vi "VariantFacade.vi"(0 "Data In":T6, 2 "Display State In":T2, 3 "Container State":T5) -> (6 "Data Out":T6, 7 "Display State Out":T2, 8 "Action":T1)   [LabVIEW 2011, in "VariantXControl__VP.xctl"]
uses:
  VariantXControl__VP.xctl
  VariantData.ctl
  <vilib>/_xctls/Container State.ctl
  VariantState.ctl
  Permissions.ctl
  TreeSettings.ctl
  <vilib>/_xctls/Action.ctl
  <userlib>/_OpenG.lib/comparison/comparison.llb/Variant Changed__ogtk.vi
  <vilib>/_xctls/XControlSupport.lvlib
panel:
  in  "VariantTree":string(tree)
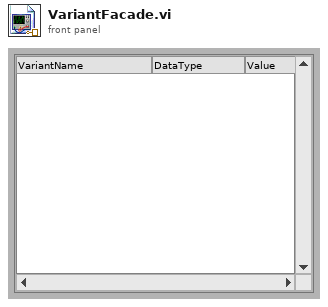
[diagram p1: front panel]
types:
  T1 = typedef "XControlSupport.lvlib/Action.ctl" = cluster{"Data Changed?":bool, "State Changed?":bool, "Action Name":string}
  T2 = typedef "VariantXControl__VP.xctl/VariantState.ctl" = cluster{"State":string, "Messages":cluster{"Message":string, "Parameter":variant}[], "Current run":i32, "Start run":i32, "LastTag":string, "Tags":string[], "Length":i32, "Permissions":T3, "IsProbe?":bool, "Changed":bool, "TreeSettings":T4, "Tree Ref":refnum<vi>}
  T3 = typedef "VariantXControl__VP.xctl/Permissions.ctl" = cluster{"Reset":bool, "TraverseAttributes":bool, "Colorize":bool}
  T4 = typedef "VariantXControl__VP.xctl/TreeSettings.ctl" = cluster{"Traverse":bool, "Colorize":bool}
  T5 = typedef "XControlSupport.lvlib/Container State.ctl" = cluster{"Indicator?":bool, "Run Mode?":bool, " Refnum":refnum<vi>}
  T6 = typedef "VariantXControl__VP.xctl/VariantData.ctl" = variant
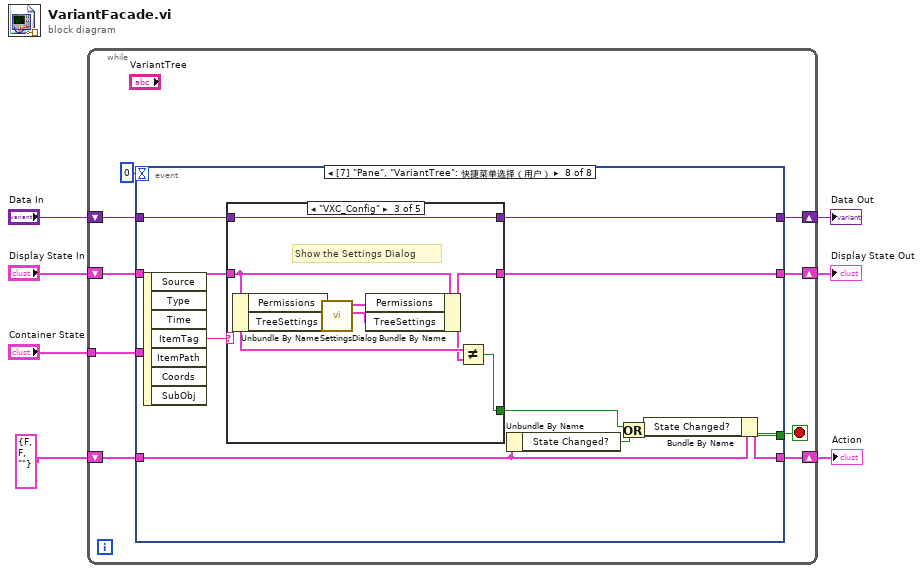
[diagram p0: block diagram]
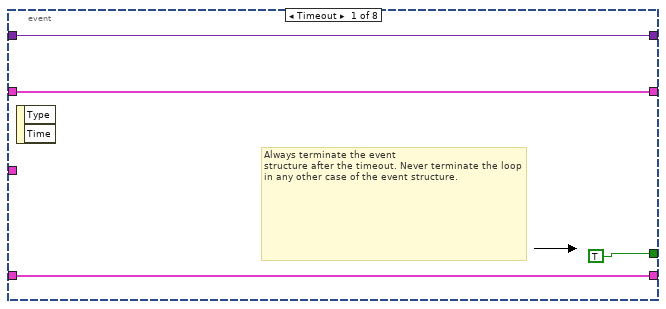
[diagram p2: hidden frame]
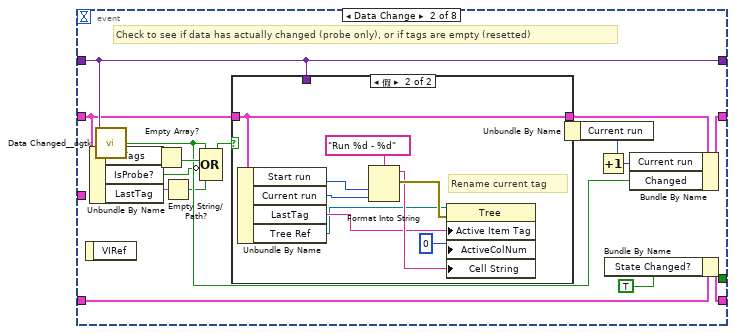
[diagram p3: hidden frame]
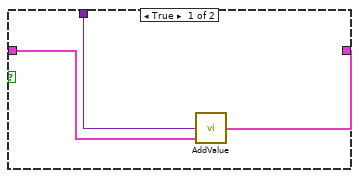
[diagram p4: hidden frame]
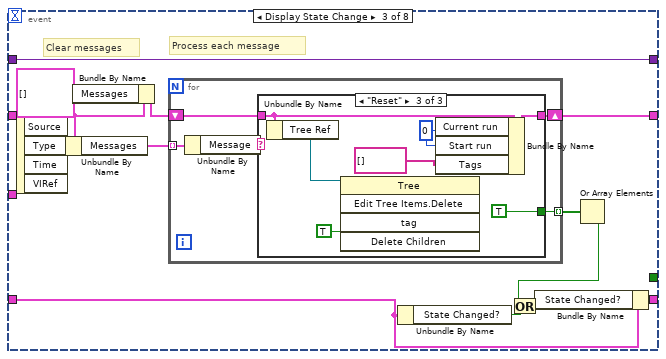
[diagram p5: hidden frame]
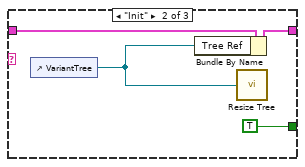
[diagram p7: hidden frame]
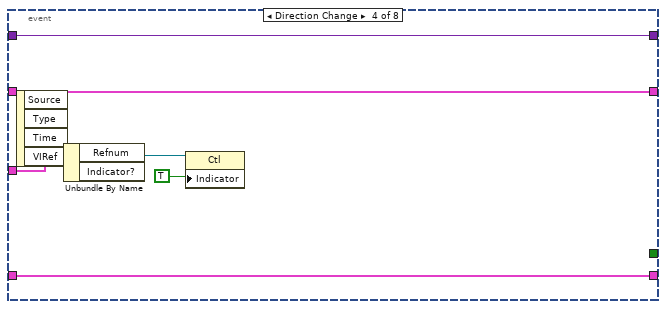
[diagram p8: hidden frame]
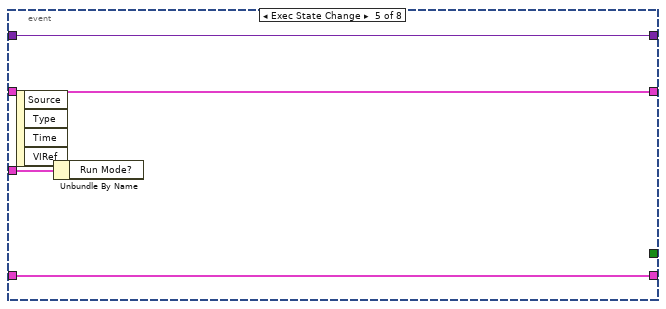
[diagram p9: hidden frame]
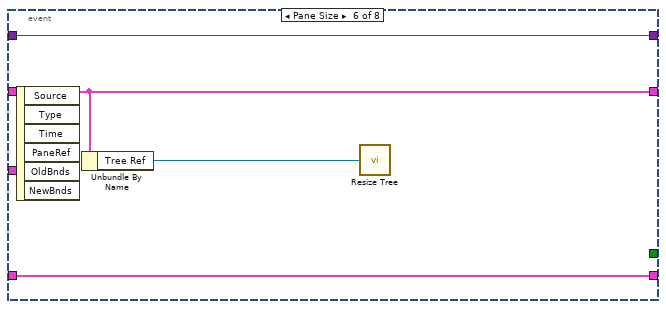
[diagram p10: hidden frame]
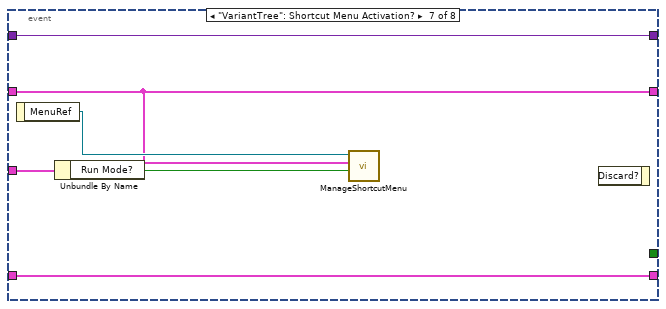
[diagram p11: hidden frame]
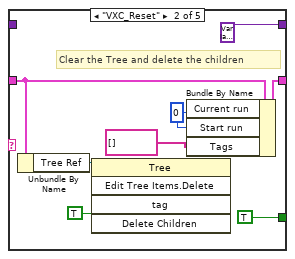
[diagram p13: hidden frame]
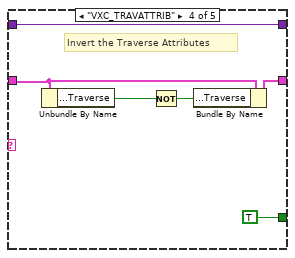
[diagram p14: hidden frame]
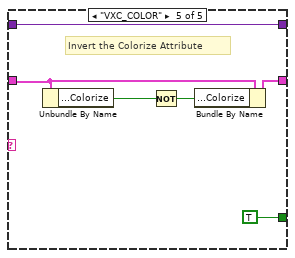
[diagram p15: hidden frame]
diagram:
  n1 = while {
    shift-right: [w15] -> w4
    shift-left: "Display State In" -> [w16]
    tunnel: "Container State" -> [w12]
    shift-right: [w10] -> w7
    shift-left: "Data In" -> [w11]
    shift-right: [w8] -> w2
    shift-left: T1 {"Data Changed?"=FALSE, "State Changed?"=FALSE, "Action Name"=""} ("Action") -> [w9]
    stop <- w14 stop-if-true
    n2 = event shown="[7] \"Pane\", \"VariantTree\": 快捷菜单选择（用户）" {
      selector: _ -> [_ _ _ _ _ _ _ _]
      dyn-events: _ -> [_ _ _ _ _ _ _ _]
      timeout: 0 -> [_ _ _ _ _ _ _ _]
      tunnel: w16 -> [w18 w28 w56 w82 w86 w89 w92 w105]
      tunnel: [w18 w31 w58 w82 w86 w89 w92 w104] -> w15
      tunnel: [TRUE _ _ _ _ _ _ _] -> w14
      tunnel: w12 -> [_ _ _ w83 w87 _ w95 _]
      tunnel: w11 -> [w17 w29 w60 w81 w85 w91 w97 w99]
      tunnel: [w17 w29 w60 w81 w85 w91 w97 w98] -> w10
      tunnel: [w19 w35 w50 w80 w84 w90 w96 w106] -> w8
      tunnel: w9 -> [w19 w36 w51 w80 w84 w90 w96 w103]
      event Timeout {
        # "Always terminate the event\nstructure after the timeout. Never terminate the loop in any other case of the event structure."
        n3 = event-data() -> ()  [unwired: 1 in, 2 out]
      }
      event Data Change {
        # "Check to see if data has actually changed (probe only), or if tags are empty (resetted)"
        n4 = event-data() -> ()  [unwired: 1 in, 1 out]
        n5 = Unbundle By Name(w28) -> ("Tags"=w27:string[], "IsProbe?"=w21:bool, "LastTag"=w23:string)
        n6 = call-poly <userlib>:"Data Changed__ogtk.vi"("Variant"=w29) -> ("Changed"=w24:bool)
        n7 = Empty Array?(array=w27) -> (empty?=w26:bool)
        n8 = Empty String/Path?(string/path=w23) -> (empty?=w22:bool)
        n9 = Compound Arithmetic op=OR(w24, w26, invert w21, w22) -> (w25:bool)
        n10 = case shown="假" w25 {
          tunnel: w28 -> [w39 w41]
          tunnel: [w38 w41] -> w32
          tunnel: w29 -> [w37 _]
          frame True {
            n11 = call "AddValue.vi"("Display State In"=w39, "Data In"=w37) -> ("Display State Out"=w38:T2)  [unwired: 1 in]
          }
          frame False {
            # "Rename current tag"
            n12 = Unbundle By Name(w41) -> ("Start run"=w45:i32, "Current run"=w42:i32, "LastTag"=w43:string, "Tree Ref"=w40:refnum<vi>)
            n13 = Format Into String(format string="Run %d - %d" ("Left Cell String"), w45, w42) -> (resulting string=w46:string, error out=w48:errorcluster)  [unwired: 2 in]
            n14 = property class="Tree"(reference=w40, error in=w48, "Active Item Tag"=w43, "ActiveColNum"=0 ("Active Cell:Active Column Number"), "Cell String"=w46) -> ()  [unwired: 2 out]
          }
        }
        n15 = Unbundle By Name(w32) -> ("Current run"=w30:i32)
        n16 = Increment(x=w30) -> (x+1=w33:i32)
        n17 = Bundle By Name(cluster=w36, "State Changed?"=TRUE) -> (w35:T1)
        n18 = Bundle By Name(cluster=w32, "Current run"=w33, "Changed"=w24) -> (w31:T2)
      }
      event Display State Change {
        # "Process each message"
        # "Clear messages"
        n19 = event-data() -> ()  [unwired: 1 in, 4 out]
        n20 = Unbundle By Name(w56) -> ("Messages"=w59:cluster{"Message":string, "Parameter":variant}[])
        n21 = Bundle By Name(cluster=w56, "Messages"=cluster{"Message":string, "Parameter":variant}[] []) -> (w55:T2)
        n22 = for {
          tunnel: w59 -> [w65] mode=indexing
          shift-right: [w62] -> w58
          shift-left: w55 -> [w63]
          tunnel: [w61] -> w57 mode=indexing
          n23 = Unbundle By Name(w65) -> ("Message"=w64:string)
          n24 = case shown="\"Reset\"" w64 {
            tunnel: w63 -> [w66 w68 w74]
            tunnel: [w66 w70 w77] -> w62
            tunnel: [_ TRUE TRUE] -> w61
            frame Default {
            }
            frame "Init" {
              n25 = control-ref of="VariantTree"() -> (w67:refnum<vi>)
              n26 = Bundle By Name(cluster=w68, "Tree Ref"=w67) -> (w70:T2)
              n27 = call "Resize Tree.vi"("Tree Ref"=w67) -> ()
            }
            frame "Reset" {
              w76 = 0 ("Current run")
              n28 = Unbundle By Name(w74) -> ("Tree Ref"=w71:refnum<vi>)
              n29 = invoke class="Tree" method="Edit Tree Items.Delete"(reference=w71, "Delete Children"=TRUE ("Delete Children?")) -> ()  [unwired: 3 in, 5 out]
              n30 = Bundle By Name(cluster=w74, "Current run"=w76, "Start run"=w76, "Tags"=string[] []) -> (w77:T2)
            }
          }
        }
        n31 = Unbundle By Name(w51) -> ("State Changed?"=w53:bool)
        n32 = Or Array Elements(Boolean array=w57) -> (logical OR=w49:bool)
        n33 = Or(x=w49, y=w53) -> (x .or. y?=w52:bool)
        n34 = Bundle By Name(cluster=w51, "State Changed?"=w52) -> (w50:T1)
      }
      event Direction Change {
        n35 = event-data() -> ()  [unwired: 1 in, 4 out]
        n36 = Unbundle By Name(w83) -> ("Refnum"=w79:refnum<vi>)  [unwired: 1 out]
        n37 = property class="Ctl"(reference=w79, "Indicator"=TRUE) -> ()  [unwired: 1 in, 2 out]
      }
      event Exec State Change {
        n38 = event-data() -> ()  [unwired: 1 in, 4 out]
        n39 = Unbundle By Name(w87) -> ()  [unwired: 1 out]
      }
      event Pane Size {
        n40 = event-data() -> ()  [unwired: 1 in, 6 out]
        n41 = Unbundle By Name(w89) -> ("Tree Ref"=w88:refnum<vi>)
        n42 = call "Resize Tree.vi"("Tree Ref"=w88) -> ()
      }
      event "VariantTree": Shortcut Menu Activation? {
        n43 = event-data() -> ("MenuRef"=w93:refnum<k9>)  [unwired: 1 in]
        n44 = Unbundle By Name(w95) -> ("Run Mode?"=w94:bool)
        n45 = call "ManageShortcutMenu.vi"("Run Mode?"=w94, "Display State In"=w92, "MenuRef"=w93) -> ()  [unwired: 9 in]
        n46 = event-data() -> ()  [unwired: 2 in, 1 out]
      }
      event "VariantTree": Shortcut Menu Selection (User) {
        n47 = event-data() -> ("ItemTag"=w107:string)  [unwired: 1 in, 6 out]
        n48 = case shown="\"VXC_Config\"" w107 {
          tunnel: [_ TRUE w120 TRUE TRUE] -> w102
          tunnel: w105 -> [w109 w114 w119 w129 w135]
          tunnel: [w109 w113 w118 w128 w134] -> w104
          tunnel: w99 -> [w108 _ w123 w131 w137]
          tunnel: [w108 T6 variant ("Data In") w123 w131 w137] -> w98
          frame Default {
          }
          frame "VXC_Reset" {
            w117 = 0 ("Current run")
            # "Clear the Tree and delete the children"
            n49 = Unbundle By Name(w114) -> ("Tree Ref"=w110:refnum<vi>)
            n50 = invoke class="Tree" method="Edit Tree Items.Delete"(reference=w110, "Delete Children"=TRUE ("Delete Children?")) -> ()  [unwired: 3 in, 5 out]
            n51 = Bundle By Name(cluster=w114, "Current run"=w117, "Start run"=w117, "Tags"=string[] []) -> (w113:T2)
          }
          frame "VXC_Config" {
            # "Show the Settings Dialog"
            n52 = Unbundle By Name(w119) -> ("Permissions"=w124:T3, "TreeSettings"=w122:T4)
            n53 = call "SettingsDialog.vi"("TreeSettings In"=w122, "Settings In"=w124) -> ("TreeSettings Out"=w121:T4, "Settings Out"=w125:T3)  [unwired: 8 in]
            n54 = Bundle By Name(cluster=w119, "Permissions"=w125, "TreeSettings"=w121) -> (w118:T2)
            n55 = Not Equal?(x=w119, y=w118) -> (x != y?=w120:bool)
          }
          frame "VXC_TRAVATTRIB" {
            # "Invert the Traverse Attributes"
            n56 = Unbundle By Name(w129) -> ("TreeSettings.Traverse"=w127:bool)
            n57 = Not(x=w127) -> (.not. x?=w126:bool)
            n58 = Bundle By Name(cluster=w129, "TreeSettings.Traverse"=w126) -> (w128:T2)
          }
          frame "VXC_COLOR" {
            # "Invert the Colorize Attribute"
            n59 = Unbundle By Name(w135) -> ("TreeSettings.Colorize"=w133:bool)
            n60 = Not(x=w133) -> (.not. x?=w132:bool)
            n61 = Bundle By Name(cluster=w135, "TreeSettings.Colorize"=w132) -> (w134:T2)
          }
        }
        n62 = Unbundle By Name(w103) -> ("State Changed?"=w101:bool)
        n63 = Or(x=w102, y=w101) -> (x .or. y?=w100:bool)
        n64 = Bundle By Name(cluster=w103, "State Changed?"=w100) -> (w106:T1)
      }
    }
  }
  "Display State Out" <- w4
  "Data Out" <- w7
  "Action" <- w2
